vi "Get Request Type.vi"(8 "error in (no error)":errorcluster, 11 "ToggleStream in":refnum<class "ToggleStream.lvclass">) -> (0 "error out":errorcluster, 2 "Request Type":string, 3 "ToggleStream out":refnum<class "ToggleStream.lvclass">)   [LabVIEW 2022 SP3, in "obs-websocket-lv.lvlib" / "ToggleStream.lvclass"]
uses:
  ToggleStream.lvclass
  ToggleStream.lvclass/ToggleStream.ctl
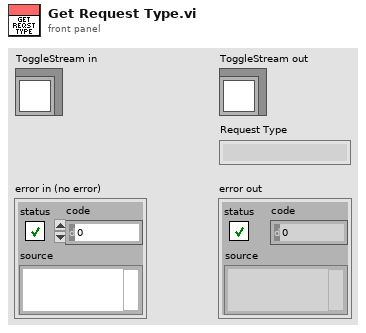
[diagram p1: front panel]
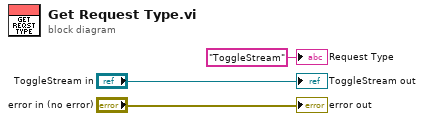
[diagram p0: block diagram]
diagram:
  "error out" <- "error in (no error)"
  "ToggleStream out" <- "ToggleStream in"
  "Request Type" <- "ToggleStream" ("Request Type")
